vi "Elevator_Execute.vi"() -> ()   [LabVIEW 2018]
uses:
  <vilib>/Rock Robotics/WPI/ThirdParty/Phoenix-LabVIEW/Motor Controller/Controls/CTRE_Phoenix_MotorControl_ControlMode.ctl
  <vilib>/Rock Robotics/WPI/Solenoid/WPI_SolenoidValue.ctl
  Global_Variables/Elevator_Globals.vi
  <vilib>/Rock Robotics/WPI/Solenoid/WPI_SolenoidGetEnum.vi
  Global_Variables/Sensor_Values.vi
  Global_Variables/Dashboard_Globals.vi
  <vilib>/Rock Robotics/WPI/Solenoid/WPI_SolenoidSetEnum.vi
panel:
  in  "Down_Limit":dbl=0.3 format="%#_13g"
  in  "Safe_Position":dbl=-1465.0
  out "Current_Position":dbl
  in  "Climb_Gain":dbl=0.00012
  in  "Down_Speed_Climb":dbl=-0.3
  in  "Up_Speed_Climb":dbl=0.25
  in  "Upper_Limit":dbl=1.0 format="%#_13g"
  in  "Gain_Down":dbl=5e-05
  in  "Gain_Up":dbl=0.0002
  in  "Gain":dbl=0.00013
  in  "Down_Gain":dbl=-1e-09
  in  "Up_Gain":dbl=-0.0013
  in  "Down_Speed":dbl=-0.25
  in  "Up_Speed":dbl=0.25
  # "1457 RPM Max speed of climb"
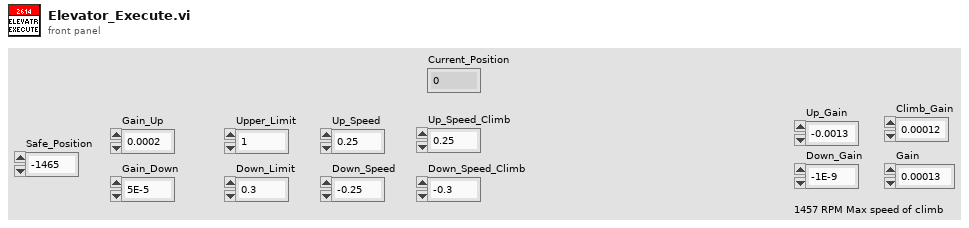
[diagram p1: front panel]
types:
  T1 = typedef "WPI_SolenoidDevRef.ctl" = cluster{"DevStatus":errorcluster, "Pneumatics Control Module":u8, "Forward Solenoid Channel":T2, "Reverse Solenoid Channel":T2}
  T2 = typedef "WPI_SolenoidChannel.ctl" = enum8{"Solenoid 0", "Solenoid 1", "Solenoid 2", "Solenoid 3", "Solenoid 4", "Solenoid 5", "Solenoid 6", "Solenoid 7", "Invalid"}
  T3 = typedef "WPI_SolenoidValue.ctl" = enum16{"Off", "On", "Forward", "Reverse"}
  T4 = typedef "WPI_MotorControlDeviceRef.ctl" = cluster{"DeviceStatus":errorcluster, "Type":T5, "PWM":cluster{"PWM Channel":T6, "DeadBand":T7}, "CAN":cluster{"Device Number":u8, "SetOutput VI Ref":variant, "GetOutput VI Ref":variant, "Enable VI Ref":variant, "Disable VI Ref":variant, "Data":variant}, "Invert":bool, "DIO PWM":cluster{"PWM \"Enable\" Channel":T6, "DIOChannel":T8, "PWM Rate":dbl}}
  T5 = typedef "WPI_MotorControlType.ctl" = enum16{"PWM", "CAN", "DIO PWM"}
  T6 = typedef "FPGA_DIOPWMChannel.ctl" = enum8{"PWM 0", "PWM 1", "PWM 2", "PWM 3", "PWM 4", "PWM 5", "PWM 6", "PWM 7", "PWM 8", "PWM 9", "PWM MXP 0", "PWM MXP 1", "PWM MXP 2", "PWM MXP 3", "PWM MXP 4", "PWM MXP 5", "PWM MXP 6", "PWM MXP 7", "PWM MXP 8", "PWM MXP 9", "Invalid"}
  T7 = typedef "WPI_PWMDeadband.ctl" = cluster{"Name":string, "maxPositivePwm":i32, "minPositivePwm":i32, "centerPwm":i32, "maxNegativePwm":i32, "minNegativePwm":i32, "angularRange":u16}
  T8 = typedef "FPGA_DIOChannel.ctl" = enum8{"DIO 0", "DIO 1", "DIO 2", "DIO 3", "DIO 4", "DIO 5", "DIO 6", "DIO 7", "DIO 8", "DIO 9", "DIO MXP 0", "DIO MXP 1", "DIO MXP 2", "DIO MXP 3", "DIO MXP 4", "DIO MXP 5", "DIO MXP 6", "DIO MXP 7", "DIO MXP 8", "DIO MXP 9", "DIO MXP 10", "DIO MXP 11", "DIO MXP 12", "DIO MXP 13", "DIO MXP 14", "DIO MXP 15", "SPI Port CS1", "SPI Port CS2", "SPI Port CS3", "SPI Port MISO", "SPI Port MOSI", "Invalid"}
  T9 = typedef "Elevator_Notifier.ctl" = cluster{"Elevator_Control_Type":T10, "Shift":bool, "Brake":bool, "Manual_Lift_Up":bool, "Manual_Lift_Down":bool, "Climb_Advance":bool, "Climb_Reverse":bool, "Low_Rocket":bool, "Mid_Rocket":bool, "High_Rocket":bool, "Cargo_Ship":bool, "Hatch_Floor":bool, "Cargo_Floor":bool, "HP_Hatch":bool, "HP_Cargo":bool, "Depot_Cargo":bool, "Stow":bool, "Set_Position":T11, "Intake_Mode":bool, "Climb_Distance":dbl, "Level_Two":bool, "Parameter_One":dbl, "Parameter_Two":dbl, "Parameter_Three":dbl, "Step":i32, "Elevator_Notifier":refnum<notifier>, "Brake_State":bool, "Shift_State":bool}
  T10 = typedef "Elevator_Control_Type.ctl" = enum16{"No_Op", "Shift", "Brake", "Manual_Elevator_Up", "Manual_Elevator_Down", "Manual_Climb_Up", "Manual_Climb_Down", "Manual_Position_Control", "Elevator_Retract", "Elevator_Extend", "Brake_In_Climb", "Position_Control", "Position", "Shift_Climb"}
  T11 = typedef "Elevator_Enum_States.ctl" = enum16{"Current_Position", "High_Rocket_Hatch_Panel_Floor", "High_Rocket_Hatch_Panel", "Mid_Rocket_Hatch_Panel_Floor", "Mid_Rocket_Hatch_Panel", "Low_Rocket_Hatch_Panel", "Cargo_Ship_Hatch_Panel", "Loading_Station_Hatch_Panel", "Ground_Pickup_Hatch_Panel", "High_Rocket_Cargo", "Mid_Rocket_Cargo", "Low_Rocket_Cargo", "Cargo_Ship_Cargo", "Loading_Station_Cargo", "Ground_Pickup_Cargo", "Depot_Pickup_Cargo", "Descend_Off_Platform", "Stow_Cargo"}
  T12 = typedef "CTRE_Phoenix_MotorControl_ControlMode.ctl" = u16
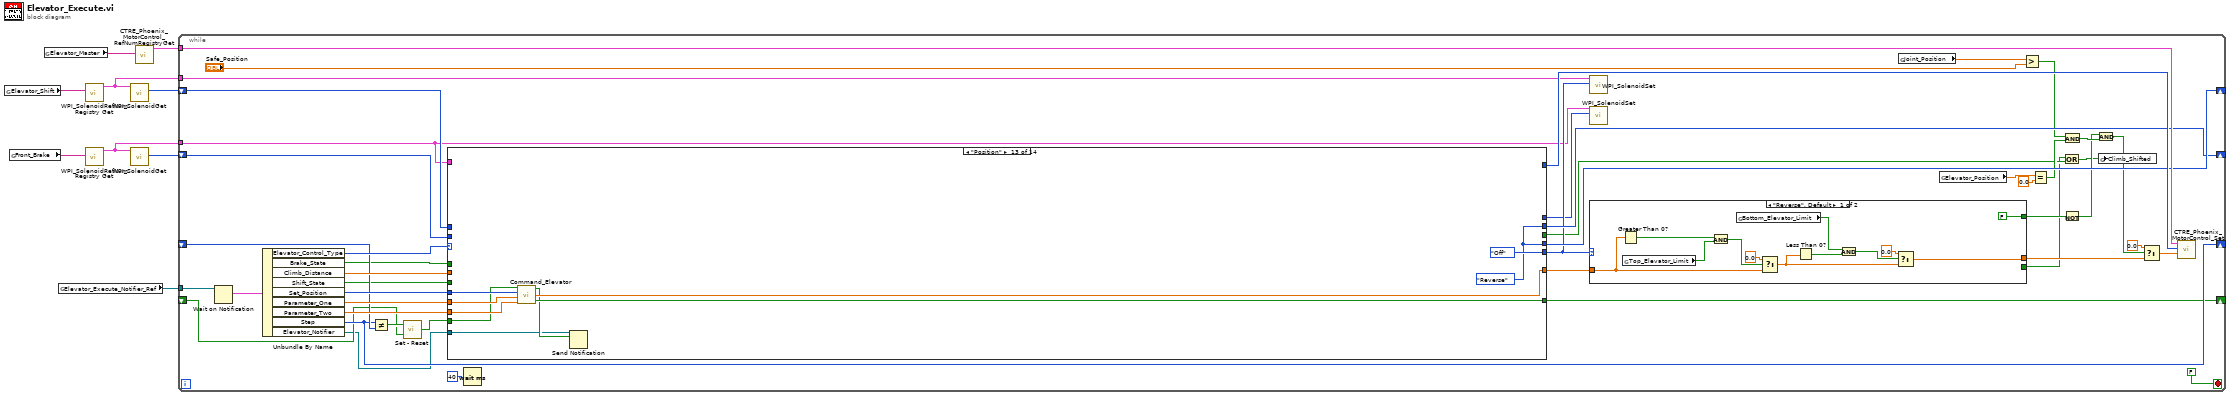
[diagram p0: block diagram]
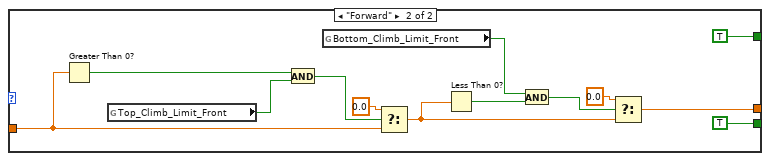
[diagram p2: hidden frame]
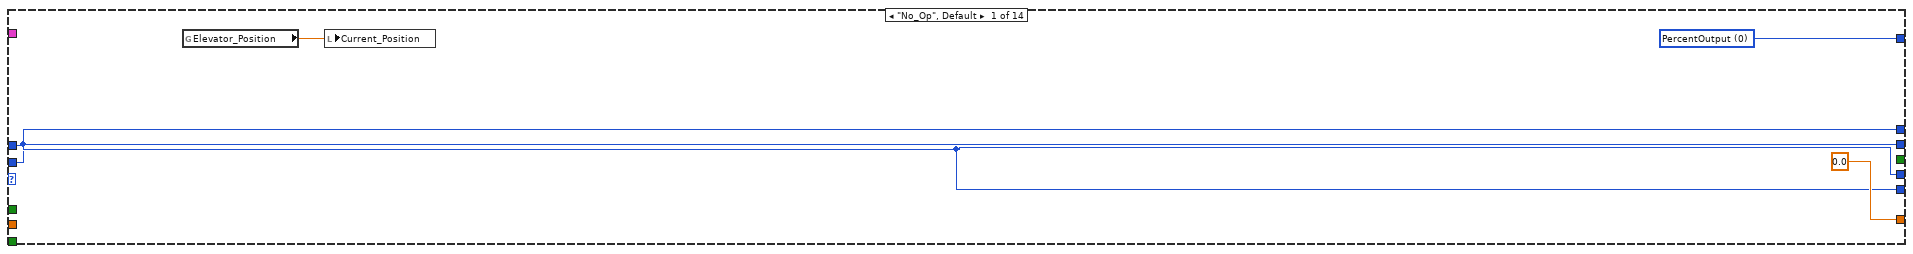
[diagram p3: hidden frame]
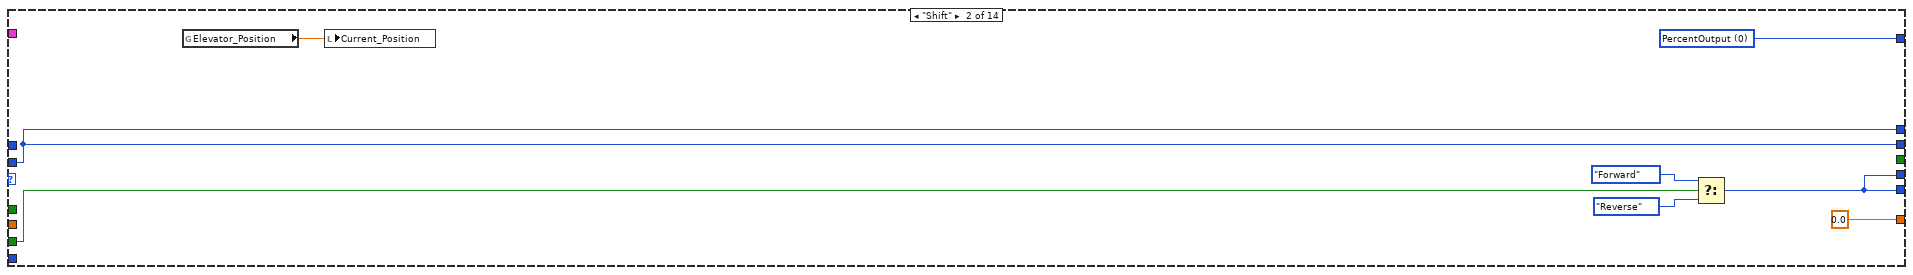
[diagram p4: hidden frame]
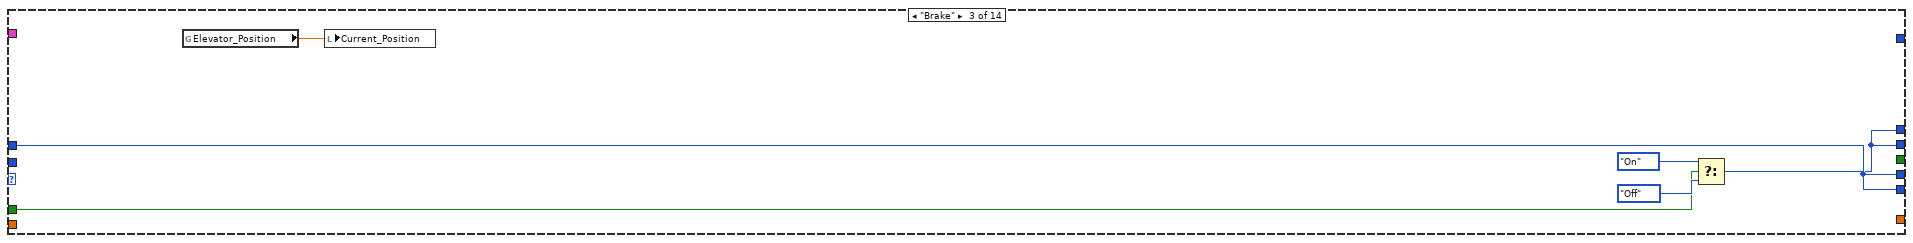
[diagram p5: hidden frame]
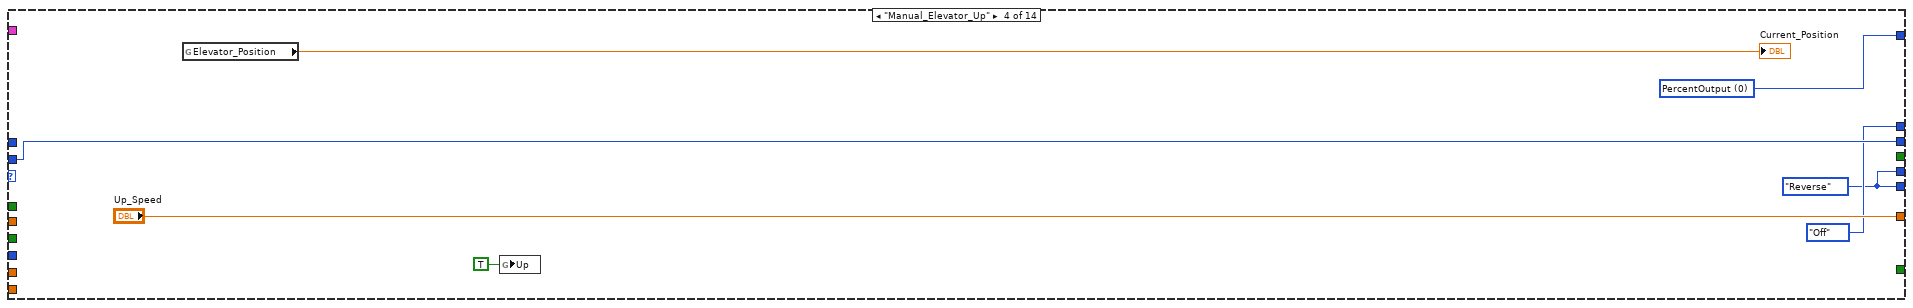
[diagram p6: hidden frame]
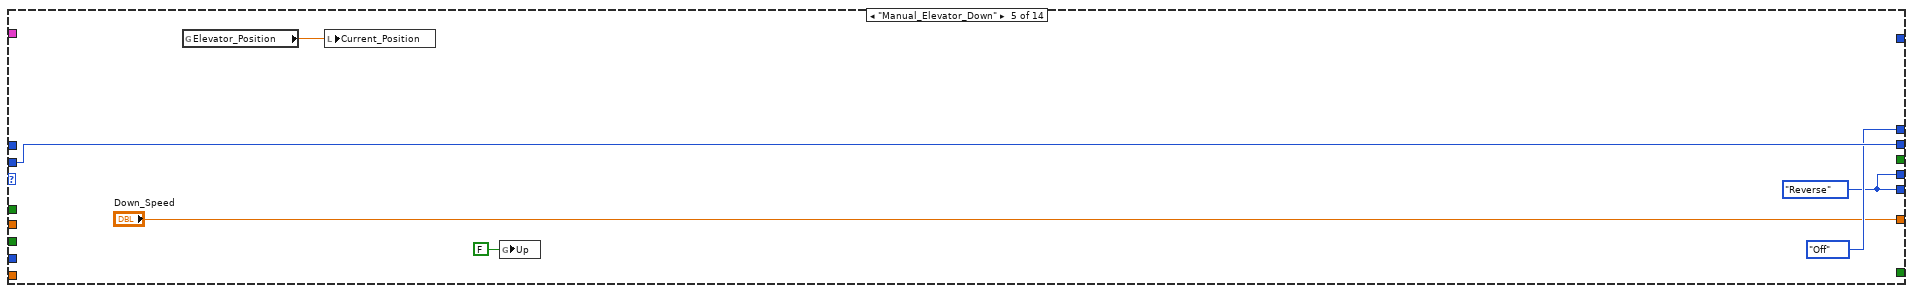
[diagram p7: hidden frame]
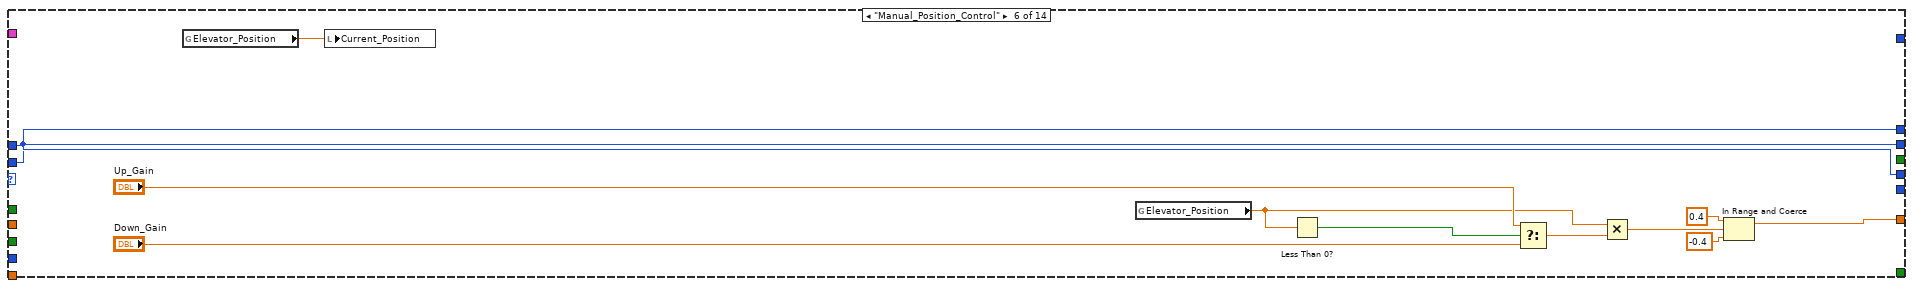
[diagram p8: hidden frame]
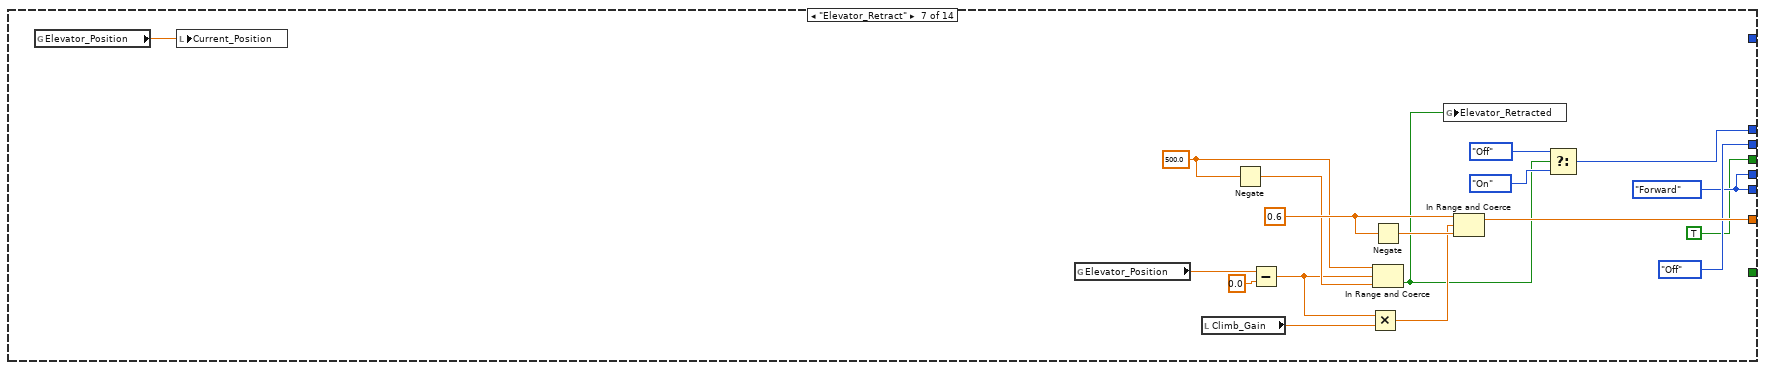
[diagram p9: hidden frame]
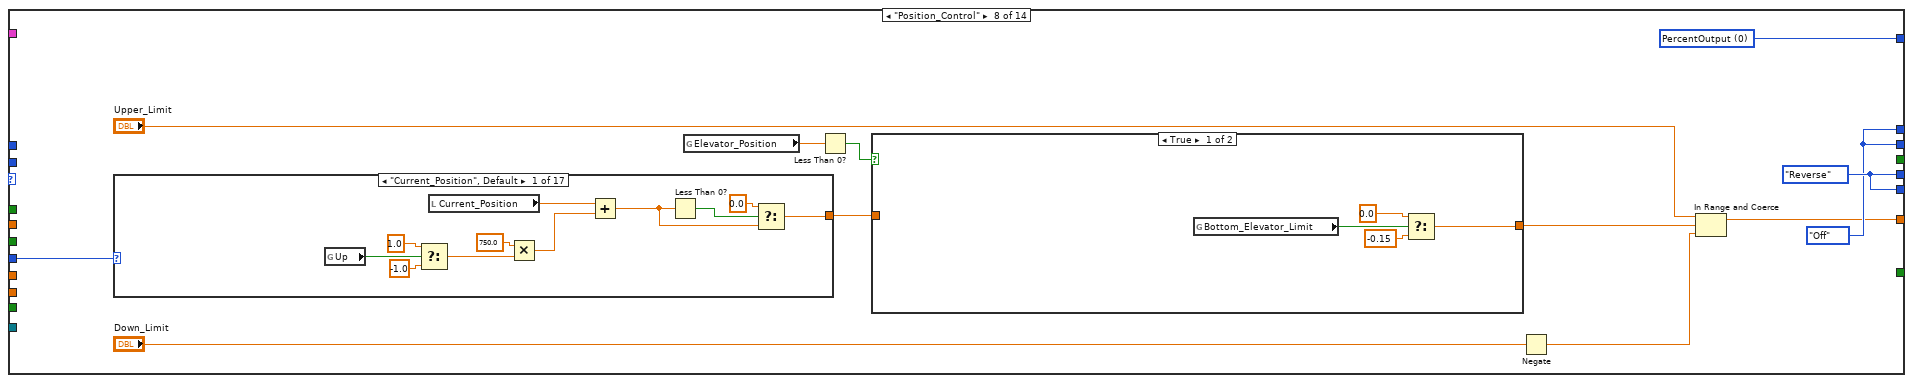
[diagram p10: hidden frame]
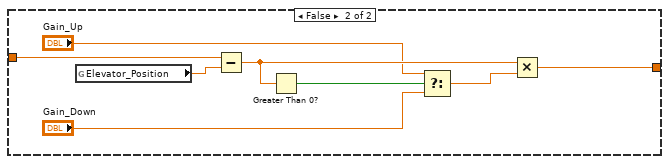
[diagram p11: hidden frame]
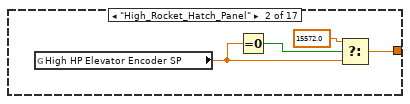
[diagram p12: hidden frame]
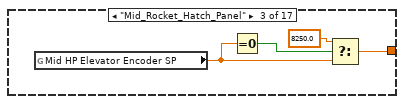
[diagram p13: hidden frame]
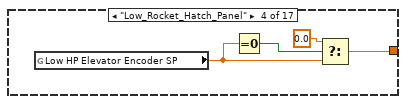
[diagram p14: hidden frame]
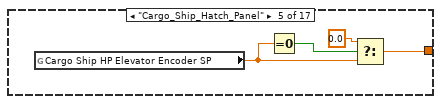
[diagram p15: hidden frame]
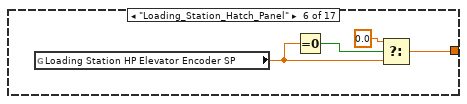
[diagram p16: hidden frame]
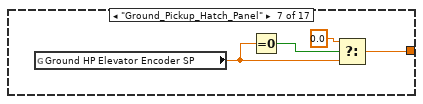
[diagram p17: hidden frame]
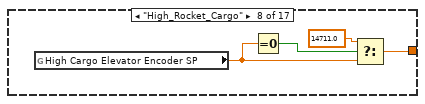
[diagram p18: hidden frame]
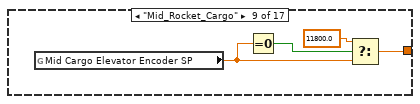
[diagram p19: hidden frame]
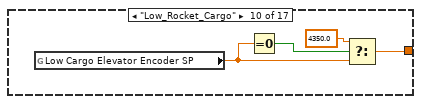
[diagram p20: hidden frame]
diagram:
  n1 = global read "Elevator_Globals.vi" "Elevator_Shift"() -> (w6:string)
  n2 = global read "Elevator_Globals.vi" "Front_Brake"() -> (w5:string)
  n3 = global read "Elevator_Globals.vi" "Elevator_Master"() -> (w7:string)
  n4 = global read "Elevator_Globals.vi" "Elevator_Execute_Notifier_Ref"() -> (w9:refnum<notifier>)
  n5 = call <vilib>:"WPI_SolenoidRefNum Registry Get.vi"("refnum name"=w6) -> ("SolenoidDevRef"=w3:T1)  [unwired: 9 in, 1 out]
  n6 = call <vilib>:"WPI_SolenoidRefNum Registry Get.vi"("refnum name"=w5) -> ("SolenoidDevRef"=w1:T1)  [unwired: 9 in, 1 out]
  n7 = call-poly <vilib>:"WPI_SolenoidGet.vi"("SolenoidDevRef"=w3) -> ("Value"=w4:T3)  [unwired: 8 in, 2 out]
  n8 = call-poly <vilib>:"WPI_SolenoidGet.vi"("SolenoidDevRef"=w1) -> ("Value"=w2:T3)  [unwired: 8 in, 2 out]
  n9 = call <vilib>:"CTRE_Phoenix_MotorControl_RefNumRegistryGet.vi"("refnum name"=w7) -> ("PhoenixMotorControlDevRef"=w8:T4)  [unwired: 9 in, 1 out]
  n10 = while {
    tunnel: w9 -> [w52]
    tunnel: w8 -> [w50]
    tunnel: w3 -> [w48]
    tunnel: w1 -> [w14]
    shift-right: [w46] -> _
    shift-left: w4 -> [w47]
    shift-right: [w45] -> _
    shift-left: w2 -> [w41]
    shift-right: [w32] -> _
    shift-left: _ -> [w33]
    shift-right: [w31] -> _
    shift-left: _ -> [w30]
    stop <- FALSE stop-if-true
    n11 = Wait on Notification(notifier=w52) -> (notification=w51:T9)  [unwired: 3 in, 3 out]
    n12 = Unbundle By Name(w51) -> ("Elevator_Control_Type"=w40:T10, "Brake_State"=w15:bool, "Climb_Distance"=w38:dbl, "Shift_State"=w13:bool, "Set_Position"=w42:T11, "Parameter_One"=w37:dbl, "Parameter_Two"=w36:dbl, "Step"=w32:i32, "Elevator_Notifier"=w29:refnum<notifier>)
    n13 = Not Equal?(x=w32, y=w33) -> (x != y?=w35:bool)
    n14 = call "Set - Reset.vi"("Reset"=w30, "Set"=w35) -> ("Output"=w34:bool)
    n15 = case shown="\"Position\"" w40 {
      tunnel: [w84 w91 _ w105 _ _ _ w153 w246 w254 _ _ _ _] -> w49
      tunnel: [0.0 ("Output") 0.0 ("Output") _ "Up_Speed" "Down_Speed" w119 w135 w147 "Up_Speed_Climb" "Down_Speed_Climb" _ w271 w293 _] -> w43
      tunnel: [w82 w88 w98 w101 w108 _ w127 w152 w245 w253 WPI_SolenoidValue."Forward" ("Value") w268 WPI_SolenoidValue."Off" ("Value") w296] -> w44
      tunnel: [w80 w87 w95 WPI_SolenoidValue."Off" ("Value") WPI_SolenoidValue."Off" ("Value") w115 w129 w151 WPI_SolenoidValue."On" ("Value") WPI_SolenoidValue."On" ("Value") WPI_SolenoidValue."Off" ("Value") w270 _ w298] -> w39
      tunnel: w47 -> [w82 _ w98 _ _ w120 _ _ _ _ w260 _ _ _]
      tunnel: [w82 w88 w98 w101 w108 w120 w127 w152 w245 w253 w260 w268 w294 w296] -> w46
      tunnel: w41 -> [w80 w87 _ w104 w111 w115 _ _ w244 w250 w259 _ _ _]
      tunnel: [w80 w87 w95 w104 w111 w115 WPI_SolenoidValue."Off" ("Value") w151 w244 w250 w259 WPI_SolenoidValue."Off" ("Value") w294 w298] -> w45
      tunnel: w13 -> [_ w85 _ _ _ _ _ _ _ _ _ _ _ _]
      tunnel: w42 -> [_ _ _ _ _ _ _ w146 _ _ _ _ w290 _]
      tunnel: w38 -> [_ _ _ _ _ _ _ _ _ _ _ w266 _ _]
      tunnel: w37 -> [_ _ _ _ _ _ _ _ _ _ _ _ w292 _]
      tunnel: w36 -> [_ _ _ _ _ _ _ _ _ _ _ _ w291 _]
      tunnel: w34 -> [_ _ _ _ _ _ _ _ _ _ _ _ w289 _]
      tunnel: [_ _ _ _ _ _ _ _ _ _ _ _ w288 _] -> w31
      tunnel: w29 -> [_ _ _ _ _ _ _ _ _ _ _ _ w286 _]
      tunnel: w14 -> [_ _ _ _ _ _ _ _ _ _ _ _ _ _]
      tunnel: w15 -> [_ _ w93 _ _ _ _ _ _ _ _ _ _ _]
      tunnel: [_ _ _ _ _ _ TRUE _ TRUE TRUE TRUE TRUE _ w297] -> w12
      frame "No_Op", Default {
        w84 = T12 0 items=["PercentOutput"=0, "Position"=1, "Velocity"=2, "Current"=3, "Follower"=5, "MotionProfile"=6, "MotionMagic"=7, "MotionProfileArc"=10, "Disabled"=15] ("Control Mode")
        n16 = global read "Sensor_Values.vi" "Elevator_Position"() -> (w81:dbl)
        n17 = local write "Current_Position"(w81) -> ()
      }
      frame "Shift" {
        w91 = T12 0 items=["PercentOutput"=0, "Position"=1, "Velocity"=2, "Current"=3, "Follower"=5, "MotionProfile"=6, "MotionMagic"=7, "MotionProfileArc"=10, "Disabled"=15] ("Control Mode")
        n18 = global read "Sensor_Values.vi" "Elevator_Position"() -> (w86:dbl)
        n19 = local write "Current_Position"(w86) -> ()
        n20 = Select(t=WPI_SolenoidValue."Forward" ("Value"), s=w85, f=WPI_SolenoidValue."Reverse" ("Value")) -> (s? t:f=w88:T3)
      }
      frame "Brake" {
        n21 = global read "Sensor_Values.vi" "Elevator_Position"() -> (w94:dbl)
        n22 = local write "Current_Position"(w94) -> ()
        n23 = Select(t=WPI_SolenoidValue."On" ("Value"), s=w93, f=WPI_SolenoidValue."Off" ("Value")) -> (s? t:f=w95:T3)
      }
      frame "Manual_Elevator_Up" {
        w101 = WPI_SolenoidValue."Reverse" ("Value")
        w105 = T12 0 items=["PercentOutput"=0, "Position"=1, "Velocity"=2, "Current"=3, "Follower"=5, "MotionProfile"=6, "MotionMagic"=7, "MotionProfileArc"=10, "Disabled"=15] ("Control Mode")
        n24 = global read "Sensor_Values.vi" "Elevator_Position"() -> (→"Current_Position":dbl)
        n25 = global write "Elevator_Globals.vi" "Up"(TRUE ("Up")) -> ()
      }
      frame "Manual_Elevator_Down" {
        w108 = WPI_SolenoidValue."Reverse" ("Value")
        n26 = global read "Sensor_Values.vi" "Elevator_Position"() -> (w107:dbl)
        n27 = local write "Current_Position"(w107) -> ()
        n28 = global write "Elevator_Globals.vi" "Up"(FALSE ("Up")) -> ()
      }
      frame "Manual_Position_Control" {
        n29 = global read "Sensor_Values.vi" "Elevator_Position"() -> (w112:dbl)
        n30 = local write "Current_Position"(w112) -> ()
        n31 = global read "Sensor_Values.vi" "Elevator_Position"() -> (w113:dbl)
        n32 = Less Than 0?(x=w113) -> (x < 0?=w114:bool)
        n33 = Select(t="Up_Gain", s=w114, f="Down_Gain") -> (s? t:f=w118:dbl)
        n34 = Multiply(x=w113, y=w118) -> (x*y=w123:dbl)
        n35 = In Range and Coerce(upper limit=0.4, x=w123, lower limit=-0.4) -> (coerced(x)=w119:dbl)  [unwired: 1 out]
      }
      frame "Elevator_Retract" {
        w131 = 500.0 ("upper limit")
        w137 = 0.6 ("upper limit")
        w127 = WPI_SolenoidValue."Forward" ("Value")
        n36 = global read "Sensor_Values.vi" "Elevator_Position"() -> (w125:dbl)
        n37 = local write "Current_Position"(w125) -> ()
        n38 = global read "Sensor_Values.vi" "Elevator_Position"() -> (w138:dbl)
        n39 = local read "Climb_Gain"() -> (w139:dbl)
        n40 = Negate(x=w131) -> (-x=w132:dbl)
        n41 = Subtract(x=w138, y=0.0) -> (x-y=w130:dbl)
        n42 = Multiply(x=w130, y=w139) -> (x*y=w140:dbl)
        n43 = Negate(x=w137) -> (-x=w141:dbl)
        n44 = In Range and Coerce(upper limit=w131, x=w130, lower limit=w132) -> (In Range?=w126:bool)  [unwired: 1 out]
        n45 = global write "Elevator_Globals.vi" "Elevator_Retracted"(w126) -> ()
        n46 = In Range and Coerce(upper limit=w137, x=w140, lower limit=w141) -> (coerced(x)=w135:dbl)  [unwired: 1 out]
        n47 = Select(t=WPI_SolenoidValue."Off" ("Value"), s=w126, f=WPI_SolenoidValue."On" ("Value")) -> (s? t:f=w129:T3)
      }
      frame "Position_Control" {
        w152 = WPI_SolenoidValue."Reverse" ("Value")
        w153 = T12 0 items=["PercentOutput"=0, "Position"=1, "Velocity"=2, "Current"=3, "Follower"=5, "MotionProfile"=6, "MotionMagic"=7, "MotionProfileArc"=10, "Disabled"=15] ("Control Mode")
        w151 = WPI_SolenoidValue."Off" ("Value")
        n48 = case shown="\"Current_Position\", Default" w146 {
          tunnel: [w175 w179 w182 w185 w190 w193 w198 w202 w206 w209 w213 w218 w222 w225 w230 w234 w237] -> w143
          frame "Current_Position", Default {
            n49 = global read "Elevator_Globals.vi" "Up"() -> (w166:bool)
            n50 = Select(t=1.0, s=w166, f=-1.0) -> (s? t:f=w170:dbl)
            n51 = local read "Current_Position"() -> (w173:dbl)
            n52 = Multiply(x=750.0 ("y"), y=w170) -> (x*y=w167:dbl)
            n53 = Add(x=w173, y=w167) -> (x+y=w172:dbl)
            n54 = Less Than 0?(x=w172) -> (x < 0?=w176:bool)
            n55 = Select(t=0.0, s=w176, f=w172) -> (s? t:f=w175:dbl)
          }
          frame "High_Rocket_Hatch_Panel" {
            n56 = global read "Dashboard_Globals.vi" "High HP Elevator Encoder SP"() -> (w178:dbl)
            n57 = Equal To 0?(x=w178) -> (x = 0?=w180:bool)
            n58 = Select(t=15572.0, s=w180, f=w178) -> (s? t:f=w179:dbl)
          }
          frame "Mid_Rocket_Hatch_Panel" {
            n59 = global read "Dashboard_Globals.vi" "Mid HP Elevator Encoder SP"() -> (w181:dbl)
            n60 = Equal To 0?(x=w181) -> (x = 0?=w184:bool)
            n61 = Select(t=8250.0, s=w184, f=w181) -> (s? t:f=w182:dbl)
          }
          frame "Low_Rocket_Hatch_Panel" {
            n62 = global read "Dashboard_Globals.vi" "Low HP Elevator Encoder SP"() -> (w186:dbl)
            n63 = Equal To 0?(x=w186) -> (x = 0?=w188:bool)
            n64 = Select(t=0.0, s=w188, f=w186) -> (s? t:f=w185:dbl)
          }
          frame "Cargo_Ship_Hatch_Panel" {
            n65 = global read "Dashboard_Globals.vi" "Cargo Ship HP Elevator Encoder SP"() -> (w189:dbl)
            n66 = Equal To 0?(x=w189) -> (x = 0?=w192:bool)
            n67 = Select(t=0.0, s=w192, f=w189) -> (s? t:f=w190:dbl)
          }
          frame "Loading_Station_Hatch_Panel" {
            n68 = global read "Dashboard_Globals.vi" "Loading Station HP Elevator Encoder SP"() -> (w194:dbl)
            n69 = Equal To 0?(x=w194) -> (x = 0?=w196:bool)
            n70 = Select(t=0.0, s=w196, f=w194) -> (s? t:f=w193:dbl)
          }
          frame "Ground_Pickup_Hatch_Panel" {
            n71 = global read "Dashboard_Globals.vi" "Ground HP Elevator Encoder SP"() -> (w197:dbl)
            n72 = Equal To 0?(x=w197) -> (x = 0?=w200:bool)
            n73 = Select(t=0.0, s=w200, f=w197) -> (s? t:f=w198:dbl)
          }
          frame "High_Rocket_Cargo" {
            n74 = global read "Dashboard_Globals.vi" "High Cargo Elevator Encoder SP"() -> (w201:dbl)
            n75 = Equal To 0?(x=w201) -> (x = 0?=w204:bool)
            n76 = Select(t=14711.0, s=w204, f=w201) -> (s? t:f=w202:dbl)
          }
          frame "Mid_Rocket_Cargo" {
            n77 = global read "Dashboard_Globals.vi" "Mid Cargo Elevator Encoder SP"() -> (w205:dbl)
            n78 = Equal To 0?(x=w205) -> (x = 0?=w208:bool)
            n79 = Select(t=11800.0, s=w208, f=w205) -> (s? t:f=w206:dbl)
          }
          frame "Low_Rocket_Cargo" {
            n80 = global read "Dashboard_Globals.vi" "Low Cargo Elevator Encoder SP"() -> (w210:dbl)
            n81 = Equal To 0?(x=w210) -> (x = 0?=w212:bool)
            n82 = Select(t=4350.0, s=w212, f=w210) -> (s? t:f=w209:dbl)
          }
          frame "Cargo_Ship_Cargo" {
            n83 = global read "Dashboard_Globals.vi" "Cargo Ship Cargo Elevator Encoder SP"() -> (w214:dbl)
            n84 = Equal To 0?(x=w214) -> (x = 0?=w216:bool)
            n85 = Select(t=7800.0, s=w216, f=w214) -> (s? t:f=w213:dbl)
          }
          frame "Loading_Station_Cargo" {
            n86 = global read "Dashboard_Globals.vi" "Loading Station Cargo Elevator Encoder SP"() -> (w217:dbl)
            n87 = Equal To 0?(x=w217) -> (x = 0?=w220:bool)
            n88 = Select(t=0.0, s=w220, f=w217) -> (s? t:f=w218:dbl)
          }
          frame "Ground_Pickup_Cargo" {
            n89 = global read "Dashboard_Globals.vi" "Ground Cargo Elevator Encoder SP"() -> (w221:dbl)
            n90 = Equal To 0?(x=w221) -> (x = 0?=w224:bool)
            n91 = Select(t=0.0, s=w224, f=w221) -> (s? t:f=w222:dbl)
          }
          frame "Depot_Pickup_Cargo" {
            n92 = global read "Dashboard_Globals.vi" "Depot Cargo Elevator Encoder SP"() -> (w226:dbl)
            n93 = Equal To 0?(x=w226) -> (x = 0?=w228:bool)
            n94 = Select(t=0.0, s=w228, f=w226) -> (s? t:f=w225:dbl)
          }
          frame "Stow_Cargo" {
            n95 = global read "Dashboard_Globals.vi" "Stow Cargo Elevator Encoder SP"() -> (w229:dbl)
            n96 = Equal To 0?(x=w229) -> (x = 0?=w232:bool)
            n97 = Select(t=0.0, s=w232, f=w229) -> (s? t:f=w230:dbl)
          }
          frame "High_Rocket_Hatch_Panel_Floor" {
            n98 = global read "Dashboard_Globals.vi" "High HP Floor Elevator Encoder SP"() -> (w233:dbl)
            n99 = Equal To 0?(x=w233) -> (x = 0?=w236:bool)
            n100 = Select(t=14000.0, s=w236, f=w233) -> (s? t:f=w234:dbl)
          }
          frame "Mid_Rocket_Hatch_Panel_Floor" {
            n101 = global read "Dashboard_Globals.vi" "Mid HP Floor Elevator Encoder SP"() -> (w238:dbl)
            n102 = Equal To 0?(x=w238) -> (x = 0?=w240:bool)
            n103 = Select(t=6300.0, s=w240, f=w238) -> (s? t:f=w237:dbl)
          }
        }
        n104 = global read "Sensor_Values.vi" "Elevator_Position"() -> (w142:dbl)
        n105 = Less Than 0?(x=w142) -> (x < 0?=w144:bool)
        n106 = case shown="True" w144 {
          tunnel: [w157 w160] -> w150
          tunnel: w143 -> [_ w158]
          frame True {
            n107 = global read "Sensor_Values.vi" "Bottom_Elevator_Limit"() -> (w156:bool)
            n108 = Select(t=0.0, s=w156, f=-0.15) -> (s? t:f=w157:dbl)
          }
          frame False {
            n109 = global read "Sensor_Values.vi" "Elevator_Position"() -> (w159:dbl)
            n110 = Subtract(x=w158, y=w159) -> (x-y=w164:dbl)
            n111 = Greater Than 0?(x=w164) -> (x > 0?=w165:bool)
            n112 = Select(t="Gain_Up", s=w165, f="Gain_Down") -> (s? t:f=w161:dbl)
            n113 = Multiply(x=w164, y=w161) -> (x*y=w160:dbl)
          }
        }
        n114 = Negate(x="Down_Limit") -> (-x=w148:dbl)
        n115 = In Range and Coerce(upper limit="Upper_Limit", x=w150, lower limit=w148) -> (coerced(x)=w147:dbl)  [unwired: 1 out]
      }
      frame "Manual_Climb_Up" {
        w245 = WPI_SolenoidValue."Forward" ("Value")
        w246 = T12 0 items=["PercentOutput"=0, "Position"=1, "Velocity"=2, "Current"=3, "Follower"=5, "MotionProfile"=6, "MotionMagic"=7, "MotionProfileArc"=10, "Disabled"=15] ("Control Mode")
        n116 = local write "Current_Position"(0.0 ("Current_Position")) -> ()
      }
      frame "Manual_Climb_Down" {
        w253 = WPI_SolenoidValue."Forward" ("Value")
        w254 = T12 0 items=["PercentOutput"=0, "Position"=1, "Velocity"=2, "Current"=3, "Follower"=5, "MotionProfile"=6, "MotionMagic"=7, "MotionProfileArc"=10, "Disabled"=15] ("Control Mode")
        n117 = local write "Current_Position"(0.0 ("Current_Position")) -> ()
      }
      frame "Brake_In_Climb" {
        n118 = global read "Sensor_Values.vi" "Elevator_Position"() -> (w256:dbl)
        n119 = local write "Current_Position"(w256) -> ()
      }
      frame "Elevator_Extend" {
        w268 = WPI_SolenoidValue."Forward" ("Value")
        w275 = 500.0 ("upper limit")
        w274 = 0.6 ("upper limit")
        n120 = local write "Current_Position"(0.0 ("Current_Position")) -> ()
        n121 = global read "Sensor_Values.vi" "Back_Climb_Position"() -> (w262:dbl)
        n122 = global read "Sensor_Values.vi" "Elevator_Position"() -> (w276:dbl)
        n123 = global read "Sensor_Values.vi" "Elevator_Position"() -> (w281:dbl)
        n124 = Negate(x=w275) -> (-x=w285:dbl)
        n125 = Subtract(x=w281, y=w266) -> (x-y=w284:dbl)
        n126 = Subtract(x=w262, y=w276) -> (x-y=w277:dbl)
        n127 = In Range and Coerce(upper limit=w275, x=w284, lower limit=w285) -> (In Range?=w267:bool)  [unwired: 1 out]
        n128 = global write "Elevator_Globals.vi" "Elevator_Extended"(w267) -> ()
        n129 = Multiply(x=w284, y="Climb_Gain") -> (x*y=w282:dbl)
        n130 = Negate(x=w274) -> (-x=w280:dbl)
        n131 = Select(t=WPI_SolenoidValue."Off" ("Value"), s=w267, f=WPI_SolenoidValue."On" ("Value")) -> (s? t:f=w270:T3)
        n132 = Multiply(x=w277, y="Gain") -> (x*y=w263:dbl)
        n133 = In Range and Coerce(upper limit=w274, x=w282, lower limit=w280) -> (coerced(x)=w279:dbl)  [unwired: 1 out]
        n134 = Negate(x=w263) -> (-x=w261:dbl)
        n135 = Add(x=w279, y=w261) -> (x+y=w271:dbl)
      }
      frame "Position" {
        w294 = WPI_SolenoidValue."Reverse" ("Value")
        n136 = call "Command_Elevator.vi"("Timeout"=w291, "Allowable_Error"=w292, "Set_Position"=w290, "Startup"=w289) -> ("Reinit"=w288:bool, "Motor_Out"=w293:dbl, "Completed"=w287:bool)
        n137 = Send Notification(notification=w287, notifier=w286) -> ()  [unwired: 1 in, 2 out]
      }
      frame "Shift_Climb" {
        w298 = WPI_SolenoidValue."Off" ("Value")
        n138 = flat-sequence {
          tunnel: [WPI_SolenoidValue."Forward" ("Value")] -> w296
          tunnel: [TRUE] -> w297
          frame #0 {
            n139 = Wait (ms)(milliseconds to wait=u32 250) -> ()  [unwired: 1 out]
          }
          frame #1 {
          }
        }
      }
    }
    n140 = Wait (ms)(milliseconds to wait=u32 40) -> ()  [unwired: 1 out]
    n141 = call-poly <vilib>:"WPI_SolenoidSet.vi"("Value"=w44, "SolenoidDevRef"=w48) -> ()  [unwired: 8 in, 2 out]
    n142 = call-poly <vilib>:"WPI_SolenoidSet.vi"("Value"=w39, "SolenoidDevRef"=w14) -> ()  [unwired: 8 in, 2 out]
    n143 = case shown="\"Reverse\", Default" w44 {
      tunnel: [w57 w70] -> w20
      tunnel: w43 -> [w56 w69]
      tunnel: [FALSE TRUE] -> w17
      tunnel: [_ TRUE] -> w10
      frame "Reverse", Default {
        n144 = Greater Than 0?(x=w56) -> (x > 0?=w66:bool)
        n145 = global read "Sensor_Values.vi" "Top_Elevator_Limit"() -> (w65:bool)
        n146 = And(x=w66, y=w65) -> (x .and. y?=w64:bool)
        n147 = global read "Sensor_Values.vi" "Bottom_Elevator_Limit"() -> (w60:bool)
        n148 = Select(t=0.0, s=w64, f=w56) -> (s? t:f=w58:dbl)
        n149 = Less Than 0?(x=w58) -> (x < 0?=w59:bool)
        n150 = And(x=w60, y=w59) -> (x .and. y?=w61:bool)
        n151 = Select(t=0.0, s=w61, f=w58) -> (s? t:f=w57:dbl)
      }
      frame "Forward" {
        n152 = Greater Than 0?(x=w69) -> (x > 0?=w79:bool)
        n153 = global read "Sensor_Values.vi" "Top_Climb_Limit_Front"() -> (w78:bool)
        n154 = And(x=w79, y=w78) -> (x .and. y?=w77:bool)
        n155 = global read "Sensor_Values.vi" "Bottom_Climb_Limit_Front"() -> (w73:bool)
        n156 = Select(t=0.0, s=w77, f=w69) -> (s? t:f=w71:dbl)
        n157 = Less Than 0?(x=w71) -> (x < 0?=w72:bool)
        n158 = And(x=w73, y=w72) -> (x .and. y?=w74:bool)
        n159 = Select(t=0.0, s=w74, f=w71) -> (s? t:f=w70:dbl)
      }
    }
    n160 = global read "Sensor_Values.vi" "Joint_Position"() -> (w28:dbl)
    n161 = global read "Sensor_Values.vi" "Elevator_Position"() -> (w25:dbl)
    n162 = Greater?(x=w28, y="Safe_Position") -> (0:w23:bool)
    n163 = Equal?(x=w25, y=0.0) -> (x = y?=w22:bool)
    n164 = Or(x=w10, y=w12) -> (x .or. y?=w11:bool)
    n165 = Not(x=w17) -> (.not. x?=w16:bool)
    n166 = And(x=w23, y=w22) -> (x .and. y?=w19:bool)
    n167 = And(x=w16, y=w19) -> (x .and. y?=w18:bool)
    n168 = global write "Elevator_Globals.vi" "Climb_Shifted"(w11) -> ()
    n169 = Select(t=0.0 ("f"), s=w18, f=w20) -> (s? t:f=w26:dbl)
    n170 = call <vilib>:"CTRE_Phoenix_MotorControl_Set.vi"("Output"=w26, "Control Mode"=w49, "PhoenixMotorControlDevRef"=w50) -> ()  [unwired: 7 in, 2 out]
  }
